vi "ManualControlL0NOGENNEW.vi"() -> ()   [LabVIEW 2012]
uses:
  <vilib>/Utility/NIReport.llb/NI_report.lvclass
  <vilib>/Utility/NIReport.llb/HTML/NI_HTML.lvclass
panel:
  in  "Sum/Maj":bool=TRUE
  in  "Ib Clip select":i32(slide)=63 scale=0.0..63.0
  in  "Clipping Select":i32(slide)=1 scale=1.0..3.0
  in  "Attenuation Select":i32(slide) scale=0.0..15.0
  in  "Delay Enable":i32(slide) scale=0.0..31.0
  in  "Channel Enable":i32(slide) scale=0.0..6.0
  in  "stop":bool
  in  "Instrument VISA in":T1={"AWG VISA"="AgilentGenerator1", "Oscilloscope  VISA "="AgilentOsciloscope", "Integration Board IP"="172.16.17.47", "connection ID"=refnum, "report out"=refnum, "report file path"=path "C:/Documents and Settings/CTA_LAB01/Desktop/L0_Asic/L0 Asic Test Data"}
  out "error out":errorcluster
  in  "error in (no error)":errorcluster
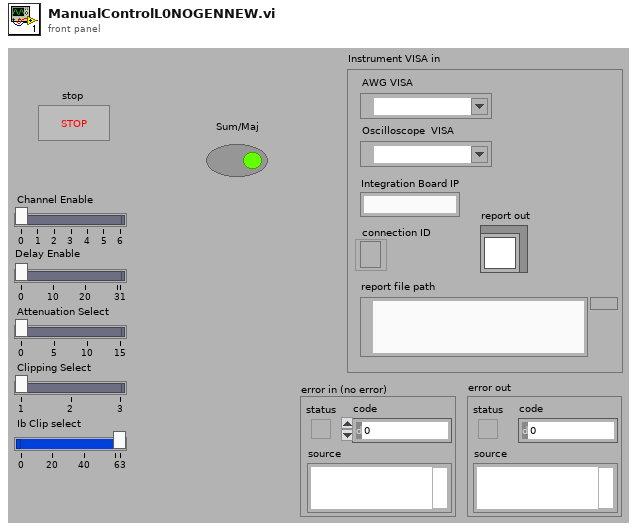
[diagram p1: front panel]
types:
  T1 = cluster{"AWG VISA":refnum<visa-resource-name>, "Oscilloscope  VISA ":refnum<visa-resource-name>, "Integration Board IP":string, "connection ID":refnum<k5>, "report out":refnum<class "NI_report.lvclass">, "report file path":path}
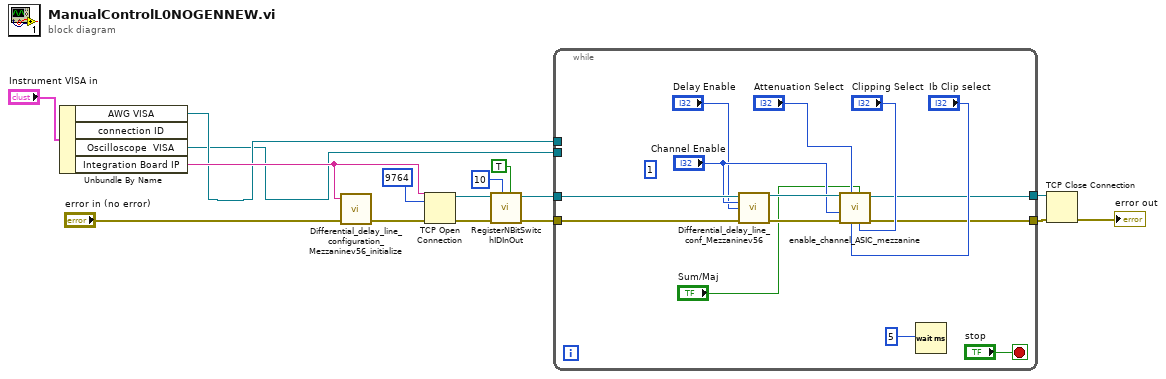
[diagram p0: block diagram]
diagram:
  n1 = Unbundle By Name("Instrument VISA in") -> ("AWG VISA"=w3:refnum<visa-resource-name>, "Oscilloscope  VISA"=w1:refnum<visa-resource-name>, "Integration Board IP"=w4:string)  [unwired: 1 out]
  n2 = call "Differential_delay_line_configuration_Mezzaninev56_initialize.vi"("error in (no error)"="error in (no error)", "address"=w4) -> ("error out 2"=w13:errorcluster)  [unwired: 1 in]
  n3 = TCP Open Connection(address=w4, remote port or service name=9764, error in (no error)=w13) -> (connection ID=w8:refnum<k5>, error out=w12:errorcluster)  [unwired: 2 in]
  n4 = call "RegisterNBitSwitchIDInOut.vi"("Switch Bit"=TRUE, "N Bit"=10, "error in (no error)"=w12, "connection ID"=w8) -> ("error out"=w9:errorcluster, "connection ID out"=w7:refnum<k5>)  [unwired: 5 in]
  n5 = while {
    tunnel: [w17] -> w11
    tunnel: [w18] -> w10
    tunnel: w1 -> [_]
    tunnel: w3 -> [_]
    tunnel: w9 -> [w19]
    tunnel: w7 -> [w30]
    stop <- "stop" stop-if-true
    (unwired) 1
    n6 = call "Differential_delay_line_conf_Mezzaninev56.vi"("connection ID"=w30, "channel"="Channel Enable", "Delay value"="Delay Enable", "error in (no error)"=w19) -> ("connection ID out"=w28:refnum<k5>, "error out 2"=w29:errorcluster)  [unwired: 4 in, 6 out]
    n7 = call "enable_channel_ASIC_mezzanine.vi"("Clip_sel_b"="Clipping Select", "maj/sum"="Sum/Maj", "Ib_clipVb"="Ib Clip select", "Att gain"="Attenuation Select", "error in"=w29, "Channel"="Channel Enable", "connection ID"=w28) -> ("error out"=w17:errorcluster, "connection ID out"=w18:refnum<k5>)  [unwired: 2 in, 1 out]
    n8 = Wait (ms)(milliseconds to wait=5) -> ()  [unwired: 1 out]
  }
  n9 = TCP Close Connection(connection ID=w10, error in (no error)=w11) -> (error out=→"error out":errorcluster)  [unwired: 1 in, 1 out]
